vi "Find SLSC Switch Custom Device by Slot Number.vi"(8 "error in":errorcluster, 10 "slot number":u32=1, 11 "slsc chassis in":T1 format="%.0x") -> (0 "error out":errorcluster, 2 "slsc switch custom device":T1=18446744073709551615 format="%.0x", 3 "slsc chassis out":T1 format="%.0x")   [LabVIEW 2020, in "SLSC Switch Scripting.lvlib"]
doc: "Returns the SLSC Switch custom device under the SLSC chassis in the specified slot number."
uses:
  SLSC Switch Scripting.lvlib
  <vilib>/NI VeriStand/Custom Device API/Custom Device Item Ref.ctl
  Shared/Constants.vi
  Dependencies.llb/SLSC Switch Shared.lvlib
  VeriStand SLSC Scripting API/VeriStand SLSC Scripting.lvlib
  <vilib>/NI VeriStand/Custom Device API/Custom Device API.lvlib
panel:
  in  "error message 2":string="The item at the specified slot number is not an SLSC Switch custom device."
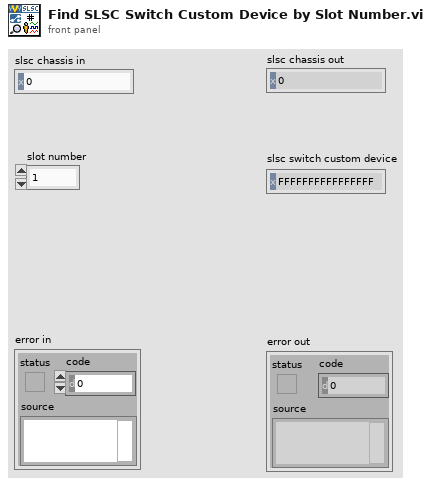
[diagram p1: front panel]
types:
  T1 = typedef "Custom Device API.lvlib/Custom Device Item Ref.ctl" = u64
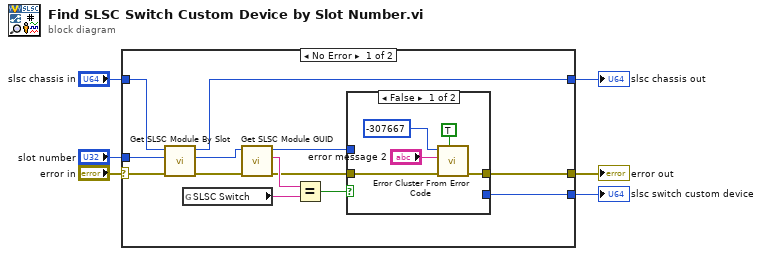
[diagram p0: block diagram]
diagram:
  n1 = case shown="No Error" "error in" {
    selector: "error in" -> [w17 w28]
    tunnel: [w16 w28] -> w5
    tunnel: "slot number" -> [w19 _]
    tunnel: [w18 _] -> w3
    tunnel: "slsc chassis in" -> [w8 w27]
    tunnel: [w7 w27] -> w1
    frame No Error {
      n2 = call "Get SLSC Module By Slot.vi"("error in (no error)"=w17, "Slot"=w19, "SLSC Chassis"=w8) -> ("error out"=w15:errorcluster, "SLSC Module"=w14:u64, "SLSC Chassis out"=w7:u64)  [unwired: 6 in]
      n3 = global read "Constants.vi" "SLSC Switch"() -> (w13:string)
      n4 = call "Get SLSC Module GUID.vi"("error in (no error)"=w15, "SLSC Module"=w14) -> ("error out"=w10:errorcluster, "Module GUID"=w11:string, "SLSC Module out"=w9:u64)  [unwired: 7 in]
      n5 = Equal?(x=w11, y=w13) -> (x = y?=w12:bool)
      n6 = case shown="False" w12 {
        tunnel: w10 -> [w23 w25]
        tunnel: [_ w26] -> w18
        tunnel: [w24 w25] -> w16
        tunnel: w9 -> [_ w26]
        frame False {
          n7 = call <vilib>:"Error Cluster From Error Code.vi"("show call chain? (False)"=TRUE, "error in (no error)"=w23, "error message (\"\")"="error message 2", "error code (0)"=-307667) -> ("error out"=w24:errorcluster)  [unwired: 5 in]
        }
        frame True {
        }
      }
    }
    frame Error {
    }
  }
  "error out" <- w5
  "slsc switch custom device" <- w3
  "slsc chassis out" <- w1
